vi "Motorgo.vi"(6 "Boolean":bool, 8 "error in (no error)":errorcluster, 9 "RightSpeed":dbl, 10 "LeftSpeed":dbl, 11 "RobotDriveDevRef 2":T1={"DevStatus"={"status"=FALSE, "code"=0, "source"=""}, "Motors[]"=[], "Square Inputs"=FALSE, "Max Output"=1.0}) -> (0 "error out":errorcluster, 2 "Motor Values":dbl[](array[numeric]), 3 "RobotDriveDevRef":T1={"DevStatus"={"status"=FALSE, "code"=0, "source"=""}, "Motors[]"=[], "Square Inputs"=FALSE, "Max Output"=1.0})   [LabVIEW 2015]
uses:
  <vilib>/Rock Robotics/WPI/RobotDrive/WPI_RobotDriveDevRef.ctl
  <vilib>/Rock Robotics/WPI/MotorControl/WPI_MotorControlDeviceRef.ctl
  <vilib>/Rock Robotics/WPI/MotorControl/WPI_MotorControlType.ctl
  <vilib>/Rock Robotics/SystemInterfaces/DIO/FPGA_DIOPWMChannel.ctl
  <vilib>/Rock Robotics/WPI/PWM/WPI_PWMDeadband.ctl
  <vilib>/Rock Robotics/WPI/CAN/Jaguar/SubVIs/WPI_CANJaguar_ControlMode.ctl
  <vilib>/Rock Robotics/WPI/CAN/TalonSRX/WPI_CANTalonSRX_APIControlMode.ctl
  <vilib>/Rock Robotics/WPI/RobotDrive/WPI_RobotDriveSafetyCheck.vi
panel:
  # "Motor Enumeration"
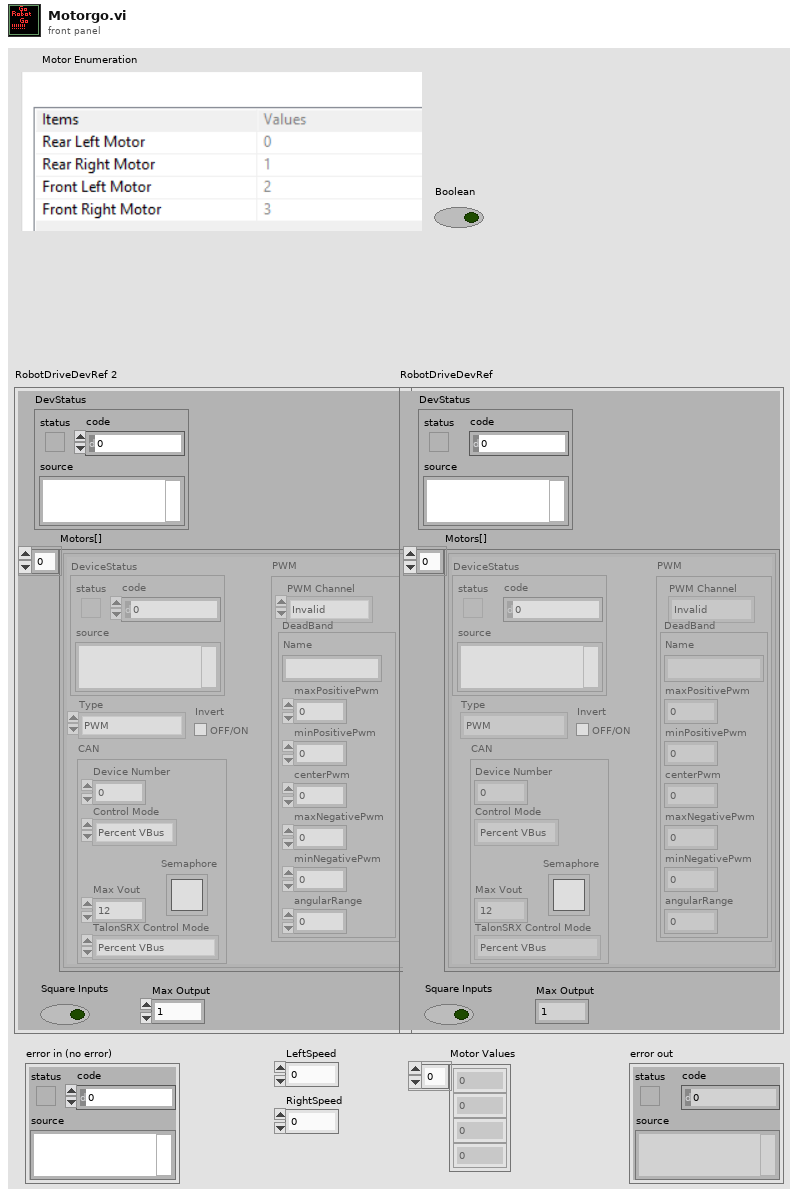
[diagram p1: front panel]
types:
  T1 = typedef "WPI_RobotDriveDevRef.ctl" = cluster{"DevStatus":errorcluster, "Motors[]":T2[], "Square Inputs":bool, "Max Output":dbl}
  T2 = typedef "WPI_MotorControlDeviceRef.ctl" = cluster{"DeviceStatus":errorcluster, "Type":T3, "PWM":cluster{"PWM Channel":T4, "DeadBand":T5}, "CAN":cluster{"Device Number":u8, "Control Mode":T6, "Semaphore":T7, "Max Vout":dbl, "TalonSRX Control Mode":T8}, "Invert":bool}
  T3 = typedef "WPI_MotorControlType.ctl" = enum16{"PWM", "CAN", "CANTalonSRX"}
  T4 = typedef "FPGA_DIOPWMChannel.ctl" = enum8{"PWM 0", "PWM 1", "PWM 2", "PWM 3", "PWM 4", "PWM 5", "PWM 6", "PWM 7", "PWM 8", "PWM 9", "PWM MXP 0", "PWM MXP 1", "PWM MXP 2", "PWM MXP 3", "PWM MXP 4", "PWM MXP 5", "PWM MXP 6", "PWM MXP 7", "PWM MXP 8", "PWM MXP 9", "Invalid"}
  T5 = typedef "WPI_PWMDeadband.ctl" = cluster{"Name":string, "maxPositivePwm":i32, "minPositivePwm":i32, "centerPwm":i32, "maxNegativePwm":i32, "minNegativePwm":i32, "angularRange":u16}
  T6 = typedef "WPI_CANJaguar_ControlMode.ctl" = enum8{"Percent VBus", "Current", "Speed", "Position", "Voltage"}
  T7 = typedef "Semaphore RefNum" = refnum<k1>
  T8 = typedef "WPI_CANTalonSRX_APIControlMode.ctl" = enum8{"Percent VBus", "Speed", "Position", "Slave", "Unchanged / Invalid", "Voltage Compensation", "Current", "Motion Profile"}
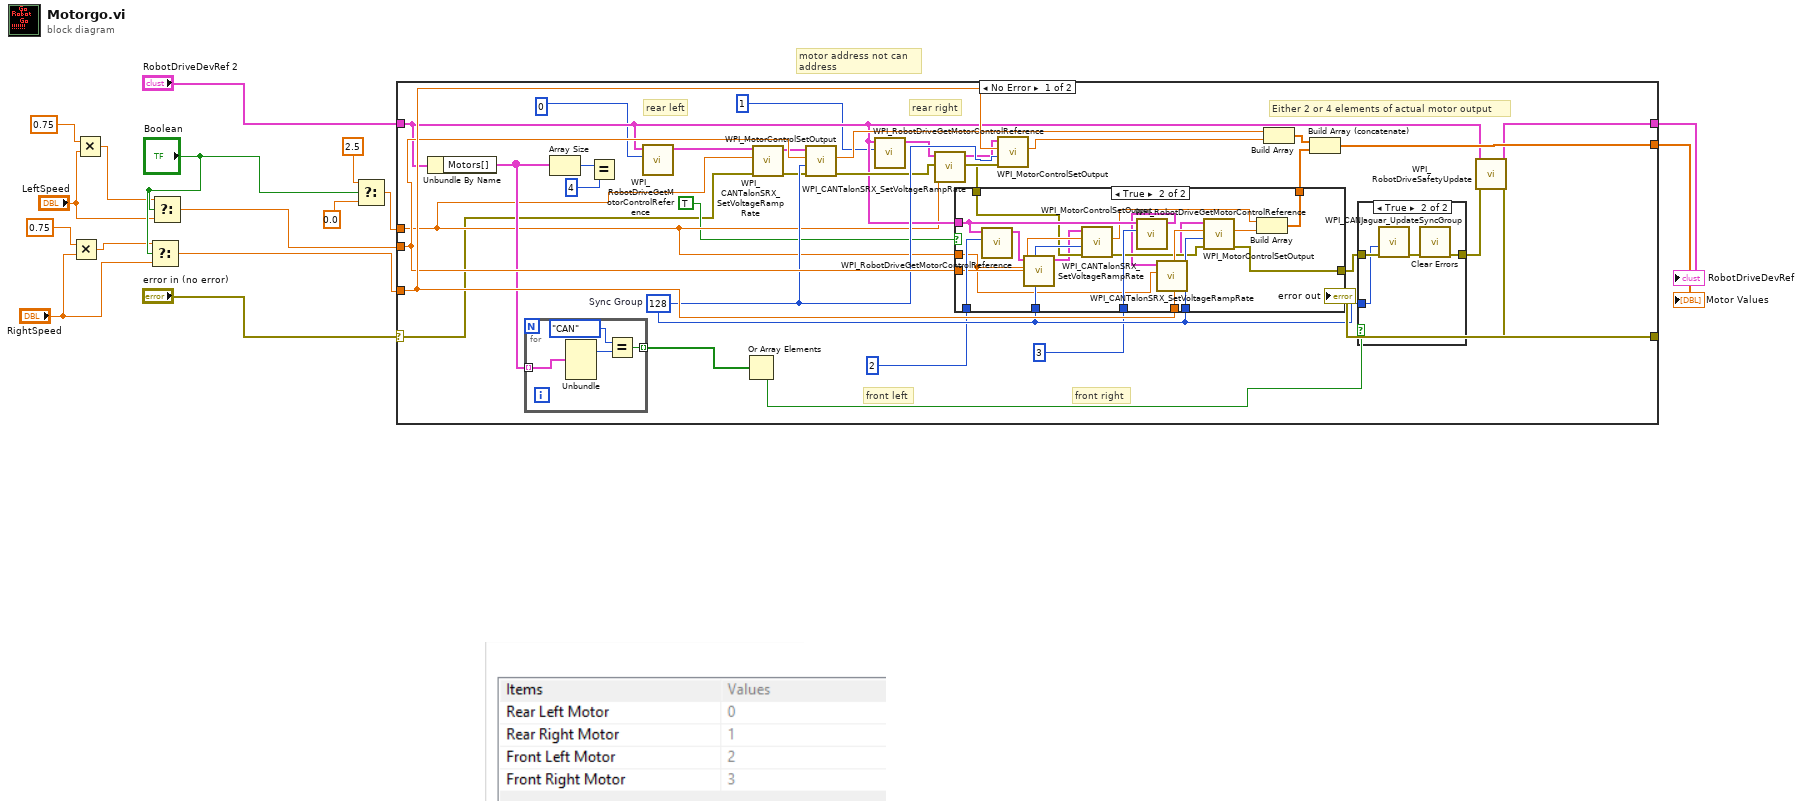
[diagram p0: block diagram]
diagram:
  # "motor address not can address"
  n1 = Multiply(x=0.75, y="RightSpeed") -> (x*y=w5:dbl)
  n2 = Multiply(x=0.75, y="LeftSpeed") -> (x*y=w3:dbl)
  n3 = Select(t=w5, s="Boolean", f="RightSpeed") -> (s? t:f=w1:dbl)
  n4 = Select(t=w3, s="Boolean", f="LeftSpeed") -> (s? t:f=w2:dbl)
  n5 = Select(t=2.5, s="Boolean", f=0.0) -> (s? t:f=w11:dbl)
  n6 = case shown="No Error" "error in (no error)" {
    selector: "error in (no error)" -> [w23 w79]
    tunnel: "RobotDriveDevRef 2" -> [w31 w78]
    tunnel: [w32 w78] -> w16
    tunnel: w2 -> [w46 _]
    tunnel: w1 -> [w47 _]
    tunnel: [w33 w79] -> w14
    tunnel: [w35 _] -> w13
    tunnel: w11 -> [w25 _]
    frame No Error {
      w45 = u8 128  # Sync Group
      # "rear left"
      # "rear right"
      # "front right"
      # "front left"
      # "Either 2 or 4 elements of actual motor output"
      n7 = Unbundle By Name(w31) -> ("Motors[]"=w44:T2[])
      n8 = for {
        tunnel: w44 -> [w53] mode=indexing
        tunnel: [w50] -> w43 mode=indexing
        n9 = Unbundle(w53) -> ("Type"=w52:T3)  [unwired: 4 out]
        n10 = Equal?(x=enum16{"PWM", "CAN"}."CAN" ("Type"), y=w52) -> (x = y?=w50:bool)
      }
      n11 = Array Size(array=w44) -> (size(s)=w49:i32)
      n12 = Equal?(x=w49, y=4) -> ()  [unwired: 1 out]
      n13 = call <vilib>:"WPI_RobotDriveGetMotorControlReference.vi"("MotorIndex"=0, "RobotDriveDevRef"=w31) -> ("MotorControlDeviceRef"=w30:T2)  [unwired: 9 out]
      n14 = Or Array Elements(Boolean array=w43) -> (logical OR=w42:bool)
      n15 = call <vilib>:"WPI_CANTalonSRX_SetVoltageRampRate.vi"("error in (no error)"=w23, "Throttle Ramp Rate (percent/s)"=w25, "CAN Talon SRX Ref"=w30) -> ("error out"=w22:errorcluster, "CAN Talon SRX Ref"=w29:T2)  [unwired: 7 in]
      n16 = call <vilib>:"WPI_MotorControlSetOutput.vi"("error in (no error)"=w22, "Sync Group / Parameter Slot"=w45, "Output"=w46, "MotorControlDevRef"=w29) -> ("error out"=w41:errorcluster, "Motor Output"=w38:dbl)  [unwired: 1 in, 5 out]
      n17 = call <vilib>:"WPI_RobotDriveGetMotorControlReference.vi"("MotorIndex"=1, "RobotDriveDevRef"=w31) -> ("MotorControlDeviceRef"=w27:T2)  [unwired: 9 out]
      n18 = call <vilib>:"WPI_CANTalonSRX_SetVoltageRampRate.vi"("Throttle Ramp Rate (percent/s)"=w25, "CAN Talon SRX Ref"=w27) -> ("CAN Talon SRX Ref"=w28:T2)  [unwired: 8 in, 1 out]
      n19 = call <vilib>:"WPI_MotorControlSetOutput.vi"("error in (no error)"=w41, "Sync Group / Parameter Slot"=w45, "Output"=w47, "MotorControlDevRef"=w28) -> ("error out"=w39:errorcluster, "Motor Output"=w26:dbl)  [unwired: 1 in, 5 out]
      n20 = case shown="True" TRUE {
        tunnel: 2 -> [_ w77]
        tunnel: 3 -> [_ w76]
        tunnel: w31 -> [_ w75]
        tunnel: w45 -> [_ w74]
        tunnel: w47 -> [_ w73]
        tunnel: w46 -> [_ w72]
        tunnel: [w59 w70] -> w40
        tunnel: w45 -> [_ w71]
        tunnel: w39 -> [w59 w68]
        tunnel: [_ w65] -> w37
        tunnel: w25 -> [_ w60]
        frame False {
        }
        frame True {
          n21 = call <vilib>:"WPI_RobotDriveGetMotorControlReference.vi"("MotorIndex"=w77, "RobotDriveDevRef"=w75) -> ("MotorControlDeviceRef"=w64:T2)  [unwired: 9 out]
          n22 = call <vilib>:"WPI_CANTalonSRX_SetVoltageRampRate.vi"("Throttle Ramp Rate (percent/s)"=w60, "CAN Talon SRX Ref"=w64) -> ("CAN Talon SRX Ref"=w63:T2)  [unwired: 8 in, 1 out]
          n23 = call <vilib>:"WPI_MotorControlSetOutput.vi"("error in (no error)"=w68, "Sync Group / Parameter Slot"=w71, "Output"=w72, "MotorControlDevRef"=w63) -> ("error out"=w69:errorcluster, "Motor Output"=w66:dbl)  [unwired: 1 in, 5 out]
          n24 = call <vilib>:"WPI_RobotDriveGetMotorControlReference.vi"("MotorIndex"=w76, "RobotDriveDevRef"=w75) -> ("MotorControlDeviceRef"=w62:T2)  [unwired: 9 out]
          n25 = call <vilib>:"WPI_CANTalonSRX_SetVoltageRampRate.vi"("Throttle Ramp Rate (percent/s)"=w60, "CAN Talon SRX Ref"=w62) -> ("CAN Talon SRX Ref"=w61:T2)  [unwired: 8 in, 1 out]
          n26 = call <vilib>:"WPI_MotorControlSetOutput.vi"("error in (no error)"=w69, "Sync Group / Parameter Slot"=w74, "Output"=w73, "MotorControlDevRef"=w61) -> ("error out"=w70:errorcluster, "Motor Output"=w67:dbl)  [unwired: 1 in, 5 out]
          n27 = Build Array(w66, w67) -> (w65:dbl[])
        }
      }
      n28 = Build Array(w38, w26) -> (w36:dbl[])
      n29 = Build Array (concatenate)(w36, w37) -> (w35:dbl[])
      n30 = case shown="True" w42 {
        tunnel: w40 -> [w54 w57]
        tunnel: w45 -> [_ w56]
        tunnel: [w54 w55] -> w34
        frame False {
        }
        frame True {
          n31 = call <vilib>:"WPI_CANJaguar_UpdateSyncGroup.vi"("error in (no error)"=w57, "Sync Group"=w56) -> ("error out"=w58:errorcluster)  [unwired: 9 out]
          n32 = call <vilib>:"Clear Errors.vi"("error in (no error)"=w58) -> ("error out"=w55:errorcluster)  [unwired: 1 in, 5 out]
        }
      }
      n33 = call <vilib>:"WPI_RobotDriveSafetyUpdate.vi"("error in (no error)"=w34, "RobotDriveDevRef"=w31) -> ("error out"=w33:errorcluster, "RobotDriveDevRef"=w32:T1)  [unwired: 8 out]
    }
    frame Error {
    }
  }
  "RobotDriveDevRef" <- w16
  "error out" <- w14
  "Motor Values" <- w13
